vi "DAQ.Read.vi"(8 "error in (no error)":errorcluster, 11 "DAQmx in":refnum<class "DAQmx.lvclass">) -> (0 "error out":errorcluster, 2 "Read":T1, 3 "DAQmx out":refnum<class "DAQmx.lvclass">)   [LabVIEW 2019]
uses:
  <resource>/objmgr/daqmx.rc
  <vilib>/DAQmx/read.llb/DAQmx Read (Analog 1D Wfm NChan NSamp).vi
  DAQmx.lvclass
  C:/user/patrick/hg/lockin.SMO/lvsrc/DAQ/DAQ.lvclass
  C:/Program Files (x86)/National Instruments/LabVIEW 2016/vi.lib/JKI/JKI SMO/SMO/SMO.lvclass
  DAQ/Typedefs/PublicEvents--DAQ.Read.ctl
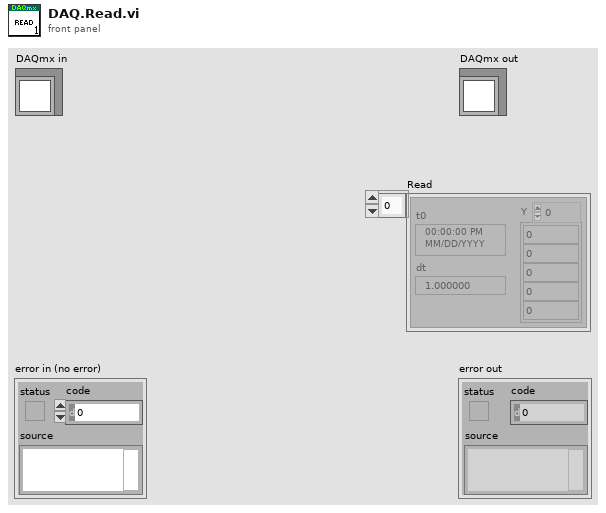
[diagram p1: front panel]
types:
  T1 = typedef "DAQ.lvclass/PublicEvents--DAQ.Read.ctl" = waveform(dbl)[]
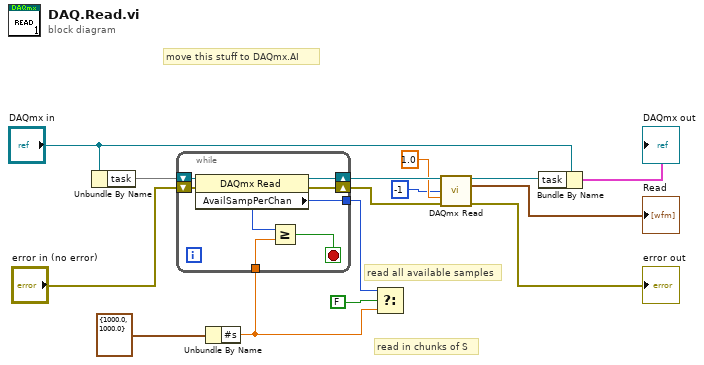
[diagram p0: block diagram]
diagram:
  # "move this stuff to DAQmx.AI"
  # "read in chunks of S"
  # "read all available samples"
  n1 = Unbundle By Name("DAQmx in") -> ("task"=w15)
  n2 = Unbundle By Name(cluster{"Fs":dbl, "#s":dbl} {"Fs"=1000.0, "#s"=1000.0} ("sampling info")) -> ("#s"=w3:dbl)
  n3 = while {
    shift-right: [w21] -> w14
    shift-left: w15 -> [w22]
    shift-right: [w20] -> w10
    shift-left: "error in (no error)" -> [w19]
    tunnel: w3 -> [w18]
    tunnel: [w16] -> w5
    stop <- w17 stop-if-true
    n4 = property class="DAQmx Read"(reference=w22, error in=w19) -> (reference out=w21:refnum<k21>, error out=w20:errorcluster, "AvailSampPerChan"=w16:u32)
    n5 = Greater Or Equal?(x=w16, y=w18) -> (x >= y?=w17:bool)
  }
  n6 = Select(t=w5, s=FALSE, f=w3) -> ()  [unwired: 1 out]
  n7 = call-poly <vilib>:"DAQmx Read.vi"("task/channels in"=w14, "number of samples per channel"=-1, "timeout"=1.0, "error in"=w10) -> ("task out"=w11:refnum<k21>, "data"=→"Read":waveform(dbl)[], "error out"=→"error out":errorcluster)  [unwired: 9 in]
  n8 = Bundle By Name(cluster="DAQmx in", "task"=w11) -> (→"DAQmx out":cluster{})
